vi "ZMC Modbus Set4x.vi"(7 "pdata":u16, 8 "error in (no error)":errorcluster caption="错误输入（无错误）", 9 "inum":u16, 10 "start":u16, 11 "handle":u32) -> (0 "error out":errorcluster caption="错误输出", 2 "function return":u32, 3 "handle out":u32, 5 "pdata out":u16)   [LabVIEW 2015, in "zauxdll.lvlib"]
doc: "uint32 __stdcall ZMC_Modbus_Set4x(ZMC_HANDLE handle, uint16 start, uint16 inum, uint16* pdata);"
uses:
  zauxdll.lvlib
  zmotion.dll
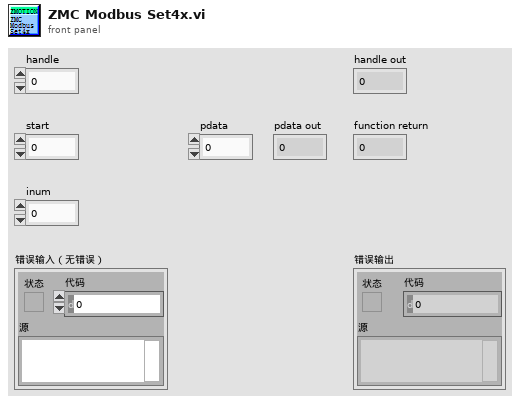
[diagram p1: front panel]
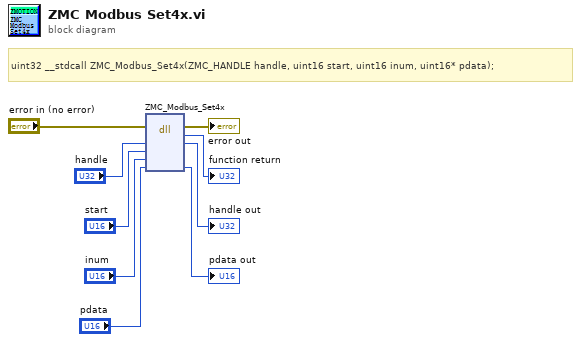
[diagram p0: block diagram]
diagram:
  # "uint32 __stdcall ZMC_Modbus_Set4x(ZMC_HANDLE handle, uint16 start, uint16 inum, uint16* pdata);"
  n1 = dll-call lib="C:/Users/VIC/Desktop/GOGORO_SA/system/LLB/zmotion/zaux/zmotion.*" fn="ZMC_Modbus_Set4x"(error in="error in (no error)", "handle"="handle", "start"="start", "inum"="inum", "pdata"="pdata") -> (error out=→"error out":errorcluster, →"function return":u32, "handle"=→"handle out":u32, "pdata"=→"pdata out":u16)  [unwired: 4 in, 1 out]
